vi "Slot Error Checker.vi"(6 "Timeout (ms)":u32=15000, 8 "error in (no error)":errorcluster, 9 "Intialize?":bool, 10 "Inputs":T1, 11 "start time":u32) -> (0 "error out":errorcluster, 4 "Slot Time":u32)   [LabVIEW 2017]
uses:
  controls/All Inputs.ctl
  controls/SACB DI.ctl
  <vilib>/ErrorRing/Error Ring.xnode
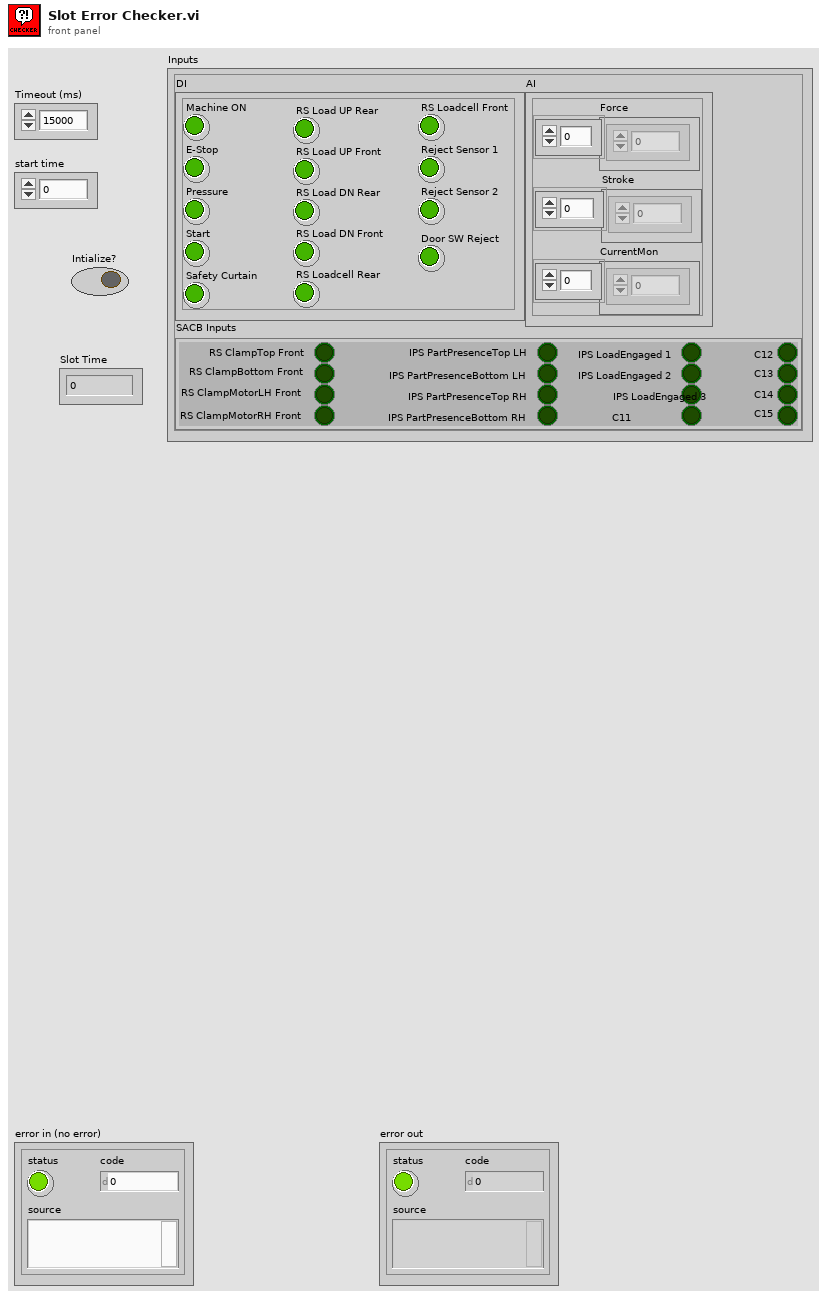
[diagram p1: front panel]
types:
  T1 = typedef "All Inputs.ctl" = cluster{"DI":cluster{"Machine ON":bool, "E-Stop":bool, "Pressure":bool, "Start":bool, "Safety Curtain":bool, "RS Load UP Rear":bool, "RS Load UP Front":bool, "RS Load DN Rear":bool, "RS Load DN Front":bool, "RS Loadcell Rear":bool, "RS Loadcell Front":bool, "Reject Sensor 1":bool, "Reject Sensor 2":bool, "Door SW Reject":bool}, "AI":cluster{"Force":dbl[], "Stroke":dbl[], "CurrentMon":dbl[]}, "SACB Inputs":T2}
  T2 = typedef "SACB DI.ctl" = cluster{"RS ClampTop Front":bool, "RS ClampBottom Front":bool, "RS ClampMotorLH Front":bool, "RS ClampMotorRH Front":bool, "IPS PartPresenceTop LH":bool, "IPS PartPresenceBottom LH":bool, "IPS PartPresenceTop RH":bool, "IPS PartPresenceBottom RH":bool, "IPS LoadEngaged 1":bool, "IPS LoadEngaged 2":bool, "IPS LoadEngaged 3":bool, "C11":bool, "C12":bool, "C13":bool, "C14":bool, "C15":bool}
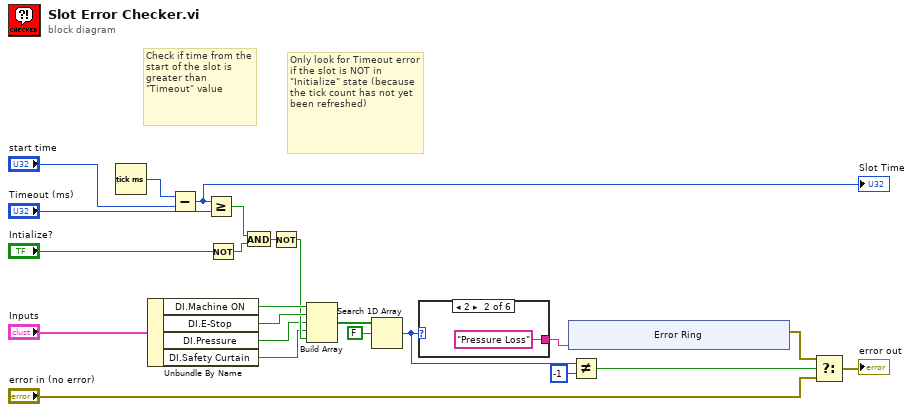
[diagram p0: block diagram]
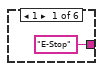
[diagram p2: hidden frame]
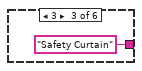
[diagram p3: hidden frame]
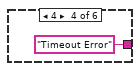
[diagram p4: hidden frame]
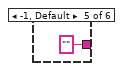
[diagram p5: hidden frame]
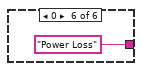
[diagram p6: hidden frame]
diagram:
  # "Only look for Timeout error if the slot is NOT in \"Initialize\" state (because the tick count has not yet been refreshed)"
  # "Check if time from the start of the slot is greater than \"Timeout\" value"
  n1 = Tick Count (ms)() -> (millisecond timer value=w17:u32)
  n2 = Unbundle By Name("Inputs") -> ("DI.Machine ON"=w5:bool, "DI.E-Stop"=w6:bool, "DI.Pressure"=w2:bool, "DI.Safety Curtain"=w1:bool)
  n3 = Subtract(x=w17, y="start time") -> (x-y=w3:u32)
  "Slot Time" <- w3
  n4 = Greater Or Equal?(x=w3, y="Timeout (ms)") -> (x >= y?=w21:bool)
  n5 = Not(x="Intialize?") -> (.not. x?=w22:bool)
  n6 = And(x=w21, y=w22) -> (x .and. y?=w23:bool)
  n7 = Not(x=w23) -> (.not. x?=w4:bool)
  n8 = Build Array(w5, w6, w2, w1, w4) -> (w7:bool[])
  n9 = Search 1D Array(1D array=w7, element=FALSE) -> (index of element=w10:i32)  [unwired: 1 in]
  n10 = case shown="2" w10 {
    tunnel: ["E-Stop" "Pressure Loss" "Safety Curtain" "Timeout Error" "" "Power Loss"] -> w9
    frame 1 {
    }
    frame 2 {
    }
    frame 3 {
    }
    frame 4 {
    }
    frame -1, Default {
    }
    frame 0 {
    }
  }
  n11 = xnode "Error Ring"("parameter 0"=w9) -> ("error out"=w13:errorcluster)
  n12 = Not Equal?(x=w10, y=-1) -> (x != y?=w12:bool)
  n13 = Select(t=w13, s=w12, f="error in (no error)") -> (s? t:f=→"error out":errorcluster)
